vi "SetAlarmControlState.vi"(8 "Error In":errorcluster, 9 "Low Limit Control Ref":refnum<vi>[](array[refnum]), 10 "High Limit Control Ref":refnum<vi>[](array[refnum]), 11 "Alarm Setups":T1[](array[typedef]) {"Low Limit (C)" format="%.1f"; "High Limit (C)" format="%.1f"}) -> (0 "Error Out":errorcluster)   [LabVIEW 2012]
uses:
  TemperatureAlarmSetup.ctl
panel:
  # "Low Limit"
  # "High Limit"
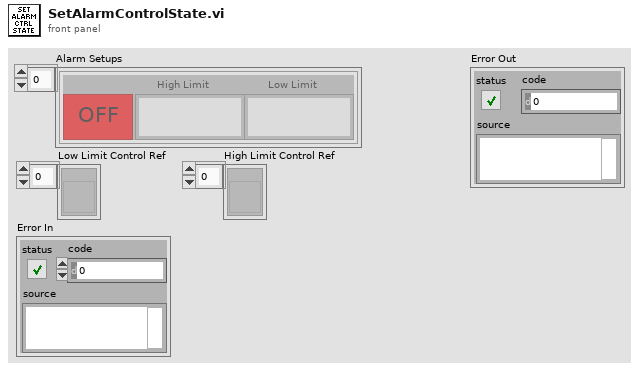
[diagram p1: front panel]
types:
  T1 = typedef "TemperatureAlarmSetup.ctl" = cluster{"ENABLED":bool, "High Limit (C)":dbl, "Low Limit (C)":dbl}
  T2 = enum8{"Enabled", "Disabled", "Disabled and Grayed Out"}
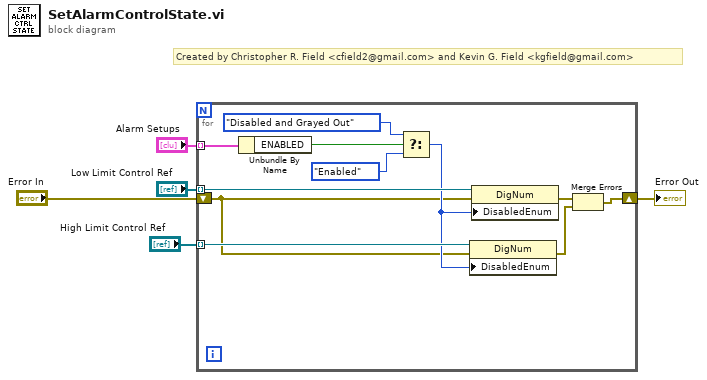
[diagram p0: block diagram]
diagram:
  # "Created by Christopher R. Field <cfield2@gmail.com> and Kevin G. Field <kgfield@gmail.com>"
  n1 = for {
    tunnel: "Alarm Setups" -> [w16] mode=indexing
    tunnel: "Low Limit Control Ref" -> [w15] mode=indexing
    shift-right: [w7] -> w3
    shift-left: "Error In" -> [w6]
    tunnel: "High Limit Control Ref" -> [w11] mode=indexing
    n2 = Unbundle By Name(w16) -> ("ENABLED"=w14:bool)
    n3 = Select(t=T2."Disabled and Grayed Out" ("Disabled"), s=w14, f=T2."Enabled" ("Disabled")) -> (s? t:f=w10:T2)
    n4 = property class="DigNum"(reference=w11, error in=w6, "DisabledEnum"=w10) -> (error out=w8:errorcluster)  [unwired: 1 out]
    n5 = property class="DigNum"(reference=w15, error in=w6, "DisabledEnum"=w10) -> (error out=w9:errorcluster)  [unwired: 1 out]
    n6 = Merge Errors(w9, w8) -> (w7:errorcluster)
  }
  "Error Out" <- w3
